vi "Fetch Single Measurement (Power).vi"(0 "VISA resource name":refnum<visa-resource-name>, 11 "error in (no error)":errorcluster) -> (2 "Power Factor":dbl, 3 "Reactive Power":dbl, 4 "VISA resource name out":refnum<visa-resource-name>, 6 "DC Power":dbl, 8 "Real Power":dbl, 10 "Apparent Power":dbl, 14 "Total Power":dbl, 15 "error out":errorcluster)   [LabVIEW 2020, in "Agilent 681x Series.lvlib"]
doc: "Fetches and returns the power measurements.\n\n<B>Note:</B>\n\nUse this VI only with other low-level VIs. The high-level VIs automatically incorporate this functionality. This VI does not check the instrument status. If you want to check the instrument status, call the Error Query VI at the conclusion of the sequence."
uses:
  <instrlib>/Agilent 681x Series/Agilent 681x Series.lvlib
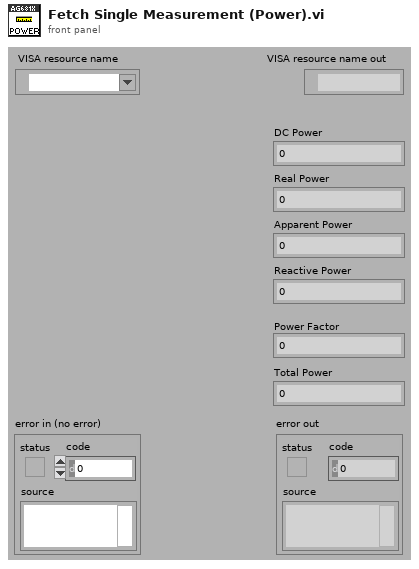
[diagram p1: front panel]
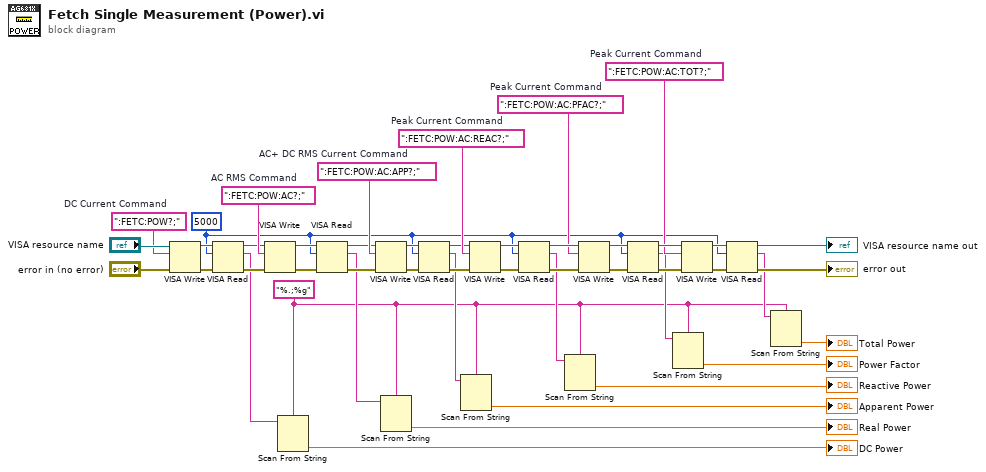
[diagram p0: block diagram]
diagram:
  w11 = ":FETC:POW:AC:TOT?;"  # Peak Current Command
  w16 = ":FETC:POW:AC:PFAC?;"  # Peak Current Command
  w1 = "%.;%g"
  w32 = ":FETC:POW:AC:REAC?;"  # Peak Current Command
  w33 = ":FETC:POW:AC:APP?;"  # AC+ DC RMS Current Command
  w41 = ":FETC:POW:AC?;"  # AC RMS Command
  w8 = u32 5000 ("byte count")
  w42 = ":FETC:POW?;"  # DC Current Command
  n1 = VISA Write(VISA resource name="VISA resource name", write buffer=w42, error in (no error)="error in (no error)") -> (VISA resource name out=w43:refnum<visa-resource-name>, error out=w44:errorcluster)  [unwired: 1 out]
  n2 = VISA Read(VISA resource name=w43, byte count=w8, error in (no error)=w44) -> (VISA resource name out=w35:refnum<visa-resource-name>, read buffer=w26:string, error out=w34:errorcluster)  [unwired: 1 out]
  n3 = VISA Write(VISA resource name=w35, write buffer=w41, error in (no error)=w34) -> (VISA resource name out=w40:refnum<visa-resource-name>, error out=w27:errorcluster)  [unwired: 1 out]
  n4 = Scan From String(format string=w1, input string=w26) -> (output 1=→"DC Power":dbl)  [unwired: 3 in, 3 out]
  n5 = VISA Read(VISA resource name=w40, byte count=w8, error in (no error)=w27) -> (VISA resource name out=w28:refnum<visa-resource-name>, read buffer=w25:string, error out=w29:errorcluster)  [unwired: 1 out]
  n6 = VISA Write(VISA resource name=w28, write buffer=w33, error in (no error)=w29) -> (VISA resource name out=w38:refnum<visa-resource-name>, error out=w39:errorcluster)  [unwired: 1 out]
  n7 = Scan From String(format string=w1, input string=w25) -> (output 1=→"Real Power":dbl)  [unwired: 3 in, 3 out]
  n8 = VISA Read(VISA resource name=w38, byte count=w8, error in (no error)=w39) -> (VISA resource name out=w31:refnum<visa-resource-name>, read buffer=w24:string, error out=w30:errorcluster)  [unwired: 1 out]
  n9 = Scan From String(format string=w1, input string=w24) -> (output 1=→"Apparent Power":dbl)  [unwired: 3 in, 3 out]
  n10 = VISA Write(VISA resource name=w31, write buffer=w32, error in (no error)=w30) -> (VISA resource name out=w37:refnum<visa-resource-name>, error out=w36:errorcluster)  [unwired: 1 out]
  n11 = VISA Read(VISA resource name=w37, byte count=w8, error in (no error)=w36) -> (VISA resource name out=w17:refnum<visa-resource-name>, read buffer=w18:string, error out=w19:errorcluster)  [unwired: 1 out]
  n12 = Scan From String(format string=w1, input string=w18) -> (output 1=→"Reactive Power":dbl)  [unwired: 3 in, 3 out]
  n13 = VISA Write(VISA resource name=w17, write buffer=w16, error in (no error)=w19) -> (VISA resource name out=w15:refnum<visa-resource-name>, error out=w14:errorcluster)  [unwired: 1 out]
  n14 = VISA Read(VISA resource name=w15, byte count=w8, error in (no error)=w14) -> (VISA resource name out=w12:refnum<visa-resource-name>, read buffer=w3:string, error out=w13:errorcluster)  [unwired: 1 out]
  n15 = Scan From String(format string=w1, input string=w3) -> (output 1=→"Power Factor":dbl)  [unwired: 3 in, 3 out]
  n16 = VISA Write(VISA resource name=w12, write buffer=w11, error in (no error)=w13) -> (VISA resource name out=w9:refnum<visa-resource-name>, error out=w10:errorcluster)  [unwired: 1 out]
  n17 = VISA Read(VISA resource name=w9, byte count=w8, error in (no error)=w10) -> (VISA resource name out=→"VISA resource name out":refnum<visa-resource-name>, read buffer=w2:string, error out=→"error out":errorcluster)  [unwired: 1 out]
  n18 = Scan From String(format string=w1, input string=w2) -> (output 1=→"Total Power":dbl)  [unwired: 3 in, 3 out]
